vi "Clear Table.vi"(7 "Confirm? (F)":bool, 8 "error in":errorcluster, 11 "Table in":refnum<vi>) -> (0 "error out":errorcluster)   [LabVIEW 2025, in "Automotive Ethernet Bus Monitor UI.lvlib"]
doc: "Clears the trace. Asks for clarification first if \"Confirm?\" is set to TRUE."
uses:
  Automotive Ethernet Bus Monitor UI.lvlib
  <vilib>/Utility/miscctls.llb/LVRowAndColumnTypeDef.ctl
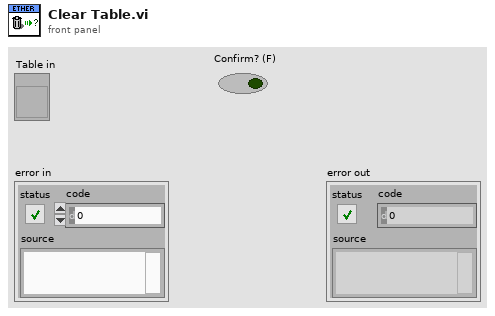
[diagram p1: front panel]
types:
  T1 = typedef "LVRowAndColumnTypeDef.ctl" = cluster{"Row":i32, "Column":i32}
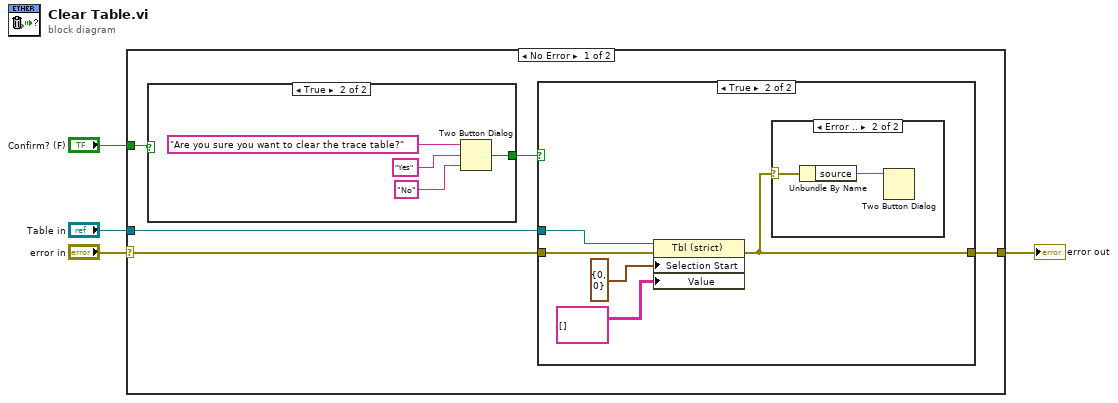
[diagram p0: block diagram]
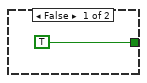
[diagram p2: hidden frame]
diagram:
  n1 = case shown="No Error" "error in" {
    selector: "error in" -> [w7 w23]
    tunnel: [w8 w23] -> w3
    tunnel: "Table in" -> [w6 _]
    tunnel: "Confirm? (F)" -> [w5 _]
    frame No Error {
      n2 = case shown="True" w5 {
        tunnel: [TRUE ("T button?") w14] -> w9
        frame False {
        }
        frame True {
          n3 = Two Button Dialog(message="Are you sure you want to clear the trace table?", 1:"No" ("F button name (\"Cancel\")"), 2:"Yes" ("T button name (\"OK\")")) -> (T button?=w14:bool)
        }
      }
      n4 = case shown="True" w9 {
        tunnel: w6 -> [_ w20]
        tunnel: [w15 w16] -> w8
        tunnel: w7 -> [w15 w17]
        frame False {
        }
        frame True {
          n5 = property class="Tbl (strict)"(reference=w20, error in=w17, "Selection Start"=T1 {"Row"=0, "Column"=0}, "Value"=string[][] [] ("Captured Data")) -> (error out=w16:errorcluster)  [unwired: 1 out]
          n6 = case shown="Error .." w16 {
            selector: w16 -> [_ w22]
            frame No Error {
            }
            frame Error {
              n7 = Unbundle By Name(w22) -> ("source"=w21:string)
              n8 = Two Button Dialog(message=w21) -> ()  [unwired: 2 in, 1 out]
            }
          }
        }
      }
    }
    frame Error {
    }
  }
  "error out" <- w3
